vi "Fit DC Hall.vi"(8 "error in":errorcluster, 10 "Data":dbl[][](array[numeric])) -> (0 "error out":errorcluster, 2 "Slope":dbl format="%#_6p", 3 "T":dbl)   [LabVIEW 2024]
panel:
  out "x/y":dbl
  out "Output file path":path
  out "Temperature":cluster{dbl[], dbl[]}(graph) caption="XY Graph"
  in  "Low field cut off":dbl=10.0
  out "Rxy(+B) - Rxy(-B)":cluster{"Binned data":dbl[], dbl[]}[](graph) caption="XY Graph"
  in  "Bin size":dbl=0.05
  in  "Save?":bool
  out "Split and binned +B and -B":cluster{dbl[], dbl[]}[](graph) caption="XY Graph"
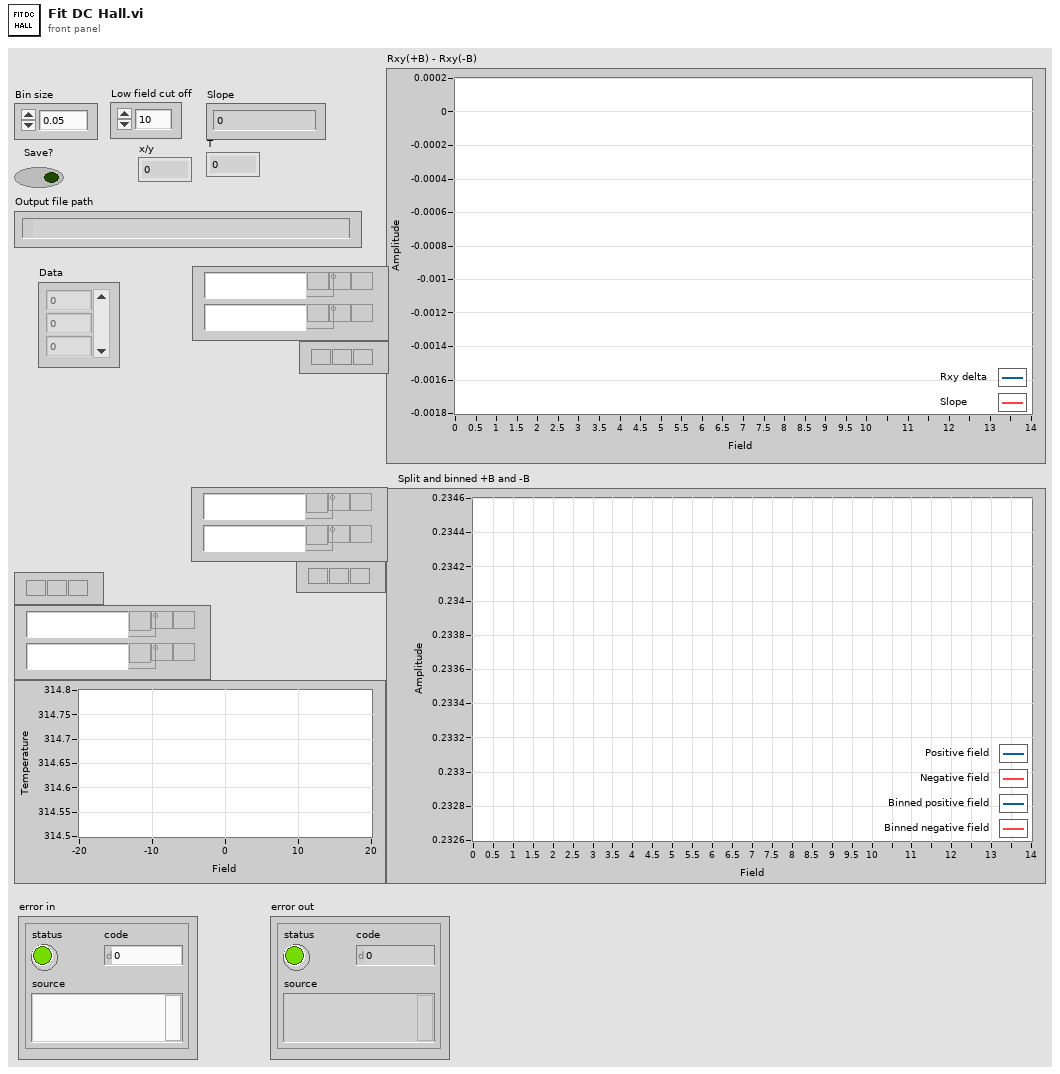
[diagram p1: front panel]
types:
  T1 = cluster{"Binned data":dbl[], "Binned data":dbl[]}
  T2 = cluster{"Output low array":dbl[], "Output low array":dbl[]}
  T3 = cluster{"Output high array":dbl[], "Output high array":dbl[]}
  T4 = cluster{"Binned data":dbl[], "Binned data":dbl[]}[]
  T5 = enum16{"open", "replace", "create", "open or create", "replace or create", "replace or create with confirmation"}
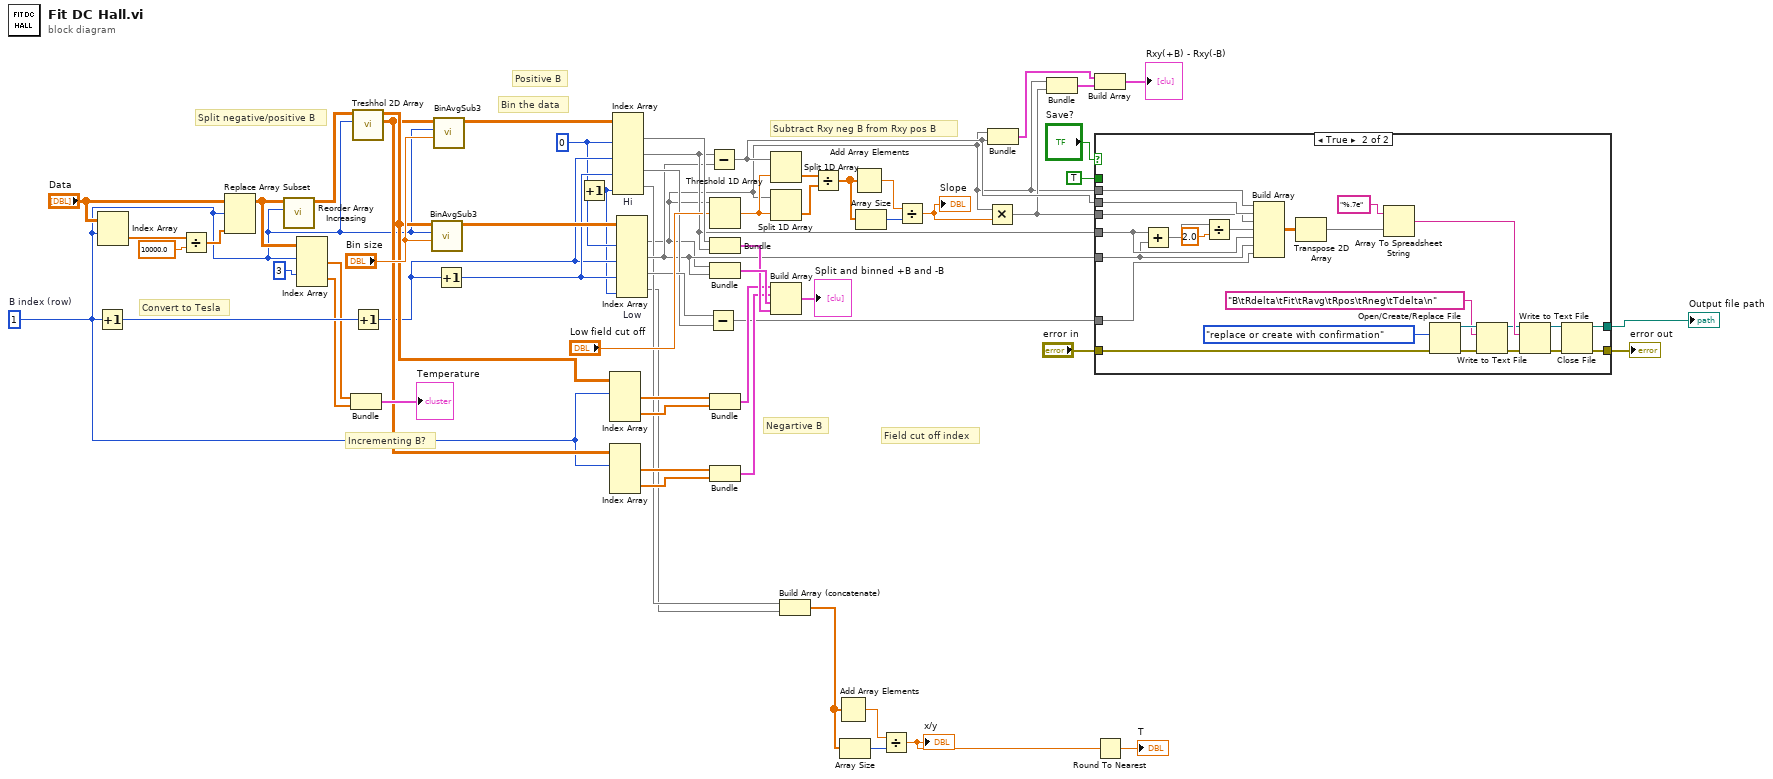
[diagram p0: block diagram]
diagram:
  w12 = 1  # B index (row)
  w10 = 0 ("disabled index (col)")
  # "Positive B"
  # "Field cut off index"
  # "Subtract Rxy neg B from Rxy pos B"
  # "Negartive B"
  # "Bin the data"
  # "Split negative/positive B"
  # "Convert to Tesla"
  # "Incrementing B?"
  n1 = Increment(x=w12) -> (x+1=w37:i32)
  n2 = Index Array(array="Data", index (row)=w12) -> (element=w29:dbl[])  [unwired: 1 in]
  n3 = Divide(x=w29, y=10000.0) -> (x/y=w28:dbl[])
  n4 = Replace Array Subset(array="Data", new element=w28, index (row)=w12) -> (w21:dbl[][])  [unwired: 1 in]
  n5 = call "Reorder Array Increasing.vi"("X row"=w12, "Array"=w21) -> ("Output array"=w31:dbl[][])  [unwired: 9 in]
  n6 = Index Array(array=w21, index (row) #1=w12, index (row) #2=3 ("index (row)")) -> (element #1=w19:dbl[], element #2=w18:dbl[])  [unwired: 2 in]
  n7 = Bundle("Data"=w19, "Data"=w18) -> (→"Temperature":cluster{"Data":dbl[], "Data":dbl[]})  [unwired: 1 in]
  n8 = call "Treshhol 2D Array.vi"("X row"=w12, "Array"=w31) -> ("Output high array"=w24:dbl[][], "Output low array"=w27:dbl[][])  [unwired: 8 in]
  n9 = Increment(x=w37) -> (x+1=w11:i32)
  n10 = call "BinAvgSub3.vi"("Bin size"="Bin size", "X coumn index"=w12, "Data in"=w27) -> ("Binned data"=w59:dbl[][])  [unwired: 2 in, 6 out]
  n11 = call "BinAvgSub3.vi"("Bin size"="Bin size", "X coumn index"=w12, "Data in"=w24) -> ("Binned data"=w58:dbl[][])  [unwired: 2 in, 6 out]
  n12 = Increment(x=w11) -> (x+1=w36:i32)
  n13 = Increment(x=w10) -> (x+1=w9:i32)
  n14 = Index Array(array=w27, index (row) #1=w12) -> (element #1=w26:dbl[], element #2=w25:dbl[])  [unwired: 3 in]
  n15 = Index Array(array=w24, index (row) #1=w12) -> (element #1=w23:dbl[], element #2=w22:dbl[])  [unwired: 3 in]
  n16 = Index Array "Hi"(array=w58, index (col) #1=w10, index (col) #2=w11, index (col) #3=w36, index (col) #4=w9) -> (element #1=w57:dbl[], element #2=w17:dbl[], element #3=w34:dbl[], element #4=w6:dbl[])  [unwired: 4 in]
  n17 = Index Array "Low"(array=w59, index (col) #1=w10, index (col) #2=w11, index (col) #3=w36, index (col) #4=w9) -> (element #1=w1:dbl[], element #2=w16:dbl[], element #3=w35:dbl[], element #4=w5:dbl[])  [unwired: 4 in]
  n18 = Subtract(x=w35, y=w34) -> (x-y=w33:dbl[])
  n19 = Subtract(x=w17, y=w16) -> (x-y=w39:dbl[])
  n20 = Threshold 1D Array(2:"Low field cut off", 3:w1) -> (0:w51:dbl)  [unwired: 1 in]
  n21 = Bundle("Binned data"=w57, "Binned data"=w17) -> (w60:T1)  [unwired: 1 in]
  n22 = Bundle("Binned data"=w1, "Binned data"=w16) -> (w62:T1)  [unwired: 1 in]
  n23 = Bundle("Output low array"=w26, "Output low array"=w25) -> (w55:T2)  [unwired: 1 in]
  n24 = Bundle("Output high array"=w23, "Output high array"=w22) -> (w54:T3)  [unwired: 1 in]
  n25 = Split 1D Array(array=w39, index=w51) -> (second subarray=w50:dbl[])  [unwired: 1 out]
  n26 = Split 1D Array(array=w1, index=w51) -> (second subarray=w49:dbl[])  [unwired: 1 out]
  n27 = Build Array(w55, w54, w62, w60) -> (→"Split and binned +B and -B":T4)
  n28 = Build Array (concatenate)(w6, w5) -> (w4:dbl[])
  n29 = Divide(x=w50, y=w49) -> (x/y=w48:dbl[])
  n30 = Add Array Elements(numeric array=w4) -> (sum=w8:dbl)
  n31 = Array Size(array=w4) -> (size(s)=w7:i32)
  n32 = Add Array Elements(numeric array=w48) -> (sum=w47:dbl)
  n33 = Array Size(array=w48) -> (size(s)=w46:i32)
  n34 = Divide(x=w8, y=w7) -> (x/y=w3:dbl)
  "x/y" <- w3
  n35 = Divide(x=w47, y=w46) -> (x/y=w45:dbl)
  "Slope" <- w45
  n36 = Multiply(x=w1, y=w45) -> (x*y=w38:dbl[])
  n37 = Bundle("Binned data"=w1, w39) -> (w53:cluster{"Binned data":dbl[], dbl[]})  [unwired: 1 in]
  n38 = Bundle("Binned data"=w1, w38) -> (w43:cluster{"Binned data":dbl[], dbl[]})  [unwired: 1 in]
  n39 = Build Array(w53, w43) -> (→"Rxy(+B) - Rxy(-B)":cluster{"Binned data":dbl[], dbl[]}[])
  n40 = case shown="True" "Save?" {
    tunnel: "error in" -> [w63 w85]
    tunnel: [w63 w72] -> w13
    tunnel: TRUE ("append to file? (new file:F)") -> [_ _]
    tunnel: w1 -> [_ w87]
    tunnel: w39 -> [_ w86]
    tunnel: w38 -> [_ w83]
    tunnel: w17 -> [_ w68]
    tunnel: w16 -> [_ w67]
    tunnel: w33 -> [_ w82]
    tunnel: [_ w70] -> w32
    frame False {
    }
    frame True {
      n41 = Add(x=w68, y=w67) -> (x+y=w66:dbl[])
      n42 = Divide(x=w66, y=2.0 ("element")) -> (x/y=w64:dbl[])
      n43 = Build Array(w87, w86, w83, w64, w68, w67, w82) -> (w79:dbl[][])
      n44 = Transpose 2D Array(2D array=w79) -> (transposed array=w78:dbl[][])
      n45 = Array To Spreadsheet String(array=w78, 3:"%.7e" ("format (%.3f)")) -> (spreadsheet string=w75:string)  [unwired: 1 in]
      n46 = Open/Create/Replace File(error in=w85, operation (0:open)=T5."replace or create with confirmation") -> (refnum out=w84:refnum<file>, error out=w80:errorcluster)  [unwired: 4 in, 1 out]
      n47 = Write to Text File(file (use dialog)=w84, text="B\tRdelta\tFit\tRavg\tRpos\tRneg\tTdelta\n", error in=w80) -> (refnum out=w74:refnum<file>, error out=w76:errorcluster)  [unwired: 1 in, 1 out]
      n48 = Write to Text File(file (use dialog)=w74, text=w75, error in=w76) -> (refnum out=w71:refnum<file>, error out=w73:errorcluster)  [unwired: 1 in, 1 out]
      n49 = Close File(refnum=w71, error in=w73) -> (path=w70:path, error out=w72:errorcluster)
    }
  }
  "Output file path" <- w32
  "error out" <- w13
  n50 = Round To Nearest(number=w3) -> (nearest integer value=→"T":dbl)
